vi "Drive_SetMotorsPosition.vi"(7 "ControlMode (CAN)":T1, 8 "error in (no error)":errorcluster, 9 "Distance Right":dbl, 10 "Distance Left":dbl) -> (0 "error out":errorcluster, 1 "Distance Right out":dbl, 2 "Distance Left out":dbl)   [LabVIEW 2009, in "Drive.lvlib"]
uses:
  Drive.lvlib
  Drive_ControlMode.ctl
  CAN/SubVIs/CAN Jaguar Control Mode.ctl
  OWNCAN.lvlib
  CAN.lvlib
  Drive_Utils.lvlib
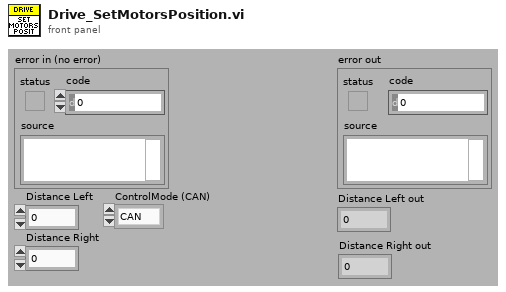
[diagram p1: front panel]
types:
  T1 = typedef "Drive.lvlib/Drive_ControlMode.ctl" = enum16{"CAN", "PWM"}
  T2 = typedef "CAN.lvlib/CAN Jaguar Control Mode.ctl" = enum16{"Percent VBus", "Speed", "Position", "Current"}
  T3 = typedef "Semaphore RefNum" = refnum<k1>
  T4 = cluster{"CAN Jaguar Ref Left":cluster{"Device Number":u8, "Control Mode":enum16{"Percent VBus", "Speed", "Position", "Current"}, "Inverted":bool, "Semaphore":T3, "Max Vout":dbl, "DevStatus":errorcluster}, "CAN Jaguar Ref Right":cluster{"Device Number":u8, "Control Mode":enum16{"Percent VBus", "Speed", "Position", "Current"}, "Inverted":bool, "Semaphore":T3, "Max Vout":dbl, "DevStatus":errorcluster}}
  T5 = enum16{"Percent VBus", "Speed", "Position", "Current"}
  T6 = typedef "OWNCAN.lvlib/CAN Jaguars Ref.ctl" = cluster{"CAN Jaguar Ref Left":T7, "CAN Jaguar Ref Right":T7}
  T7 = typedef "CAN.lvlib/CAN Jaguar Ref.ctl" = cluster{"Device Number":u8, "Control Mode":T2, "Inverted":bool, "Semaphore":T3, "Max Vout":dbl, "DevStatus":errorcluster}
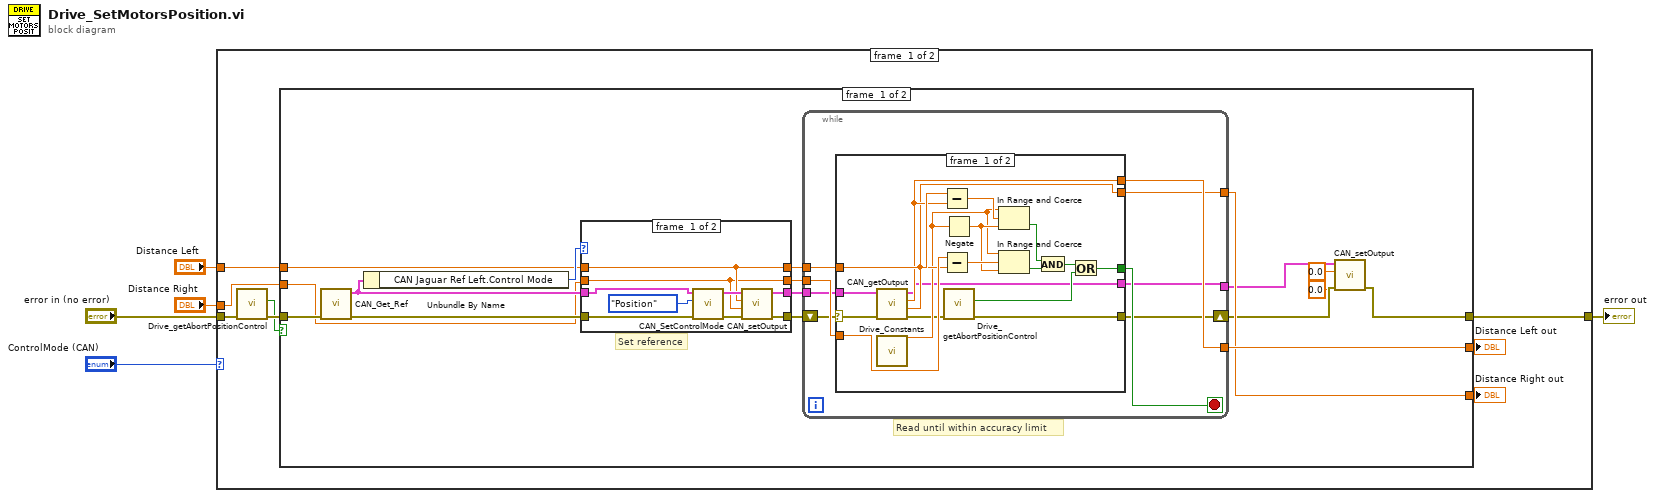
[diagram p0: block diagram]
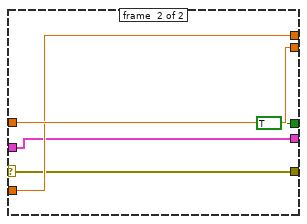
[diagram p2: hidden frame]
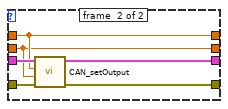
[diagram p3: hidden frame]
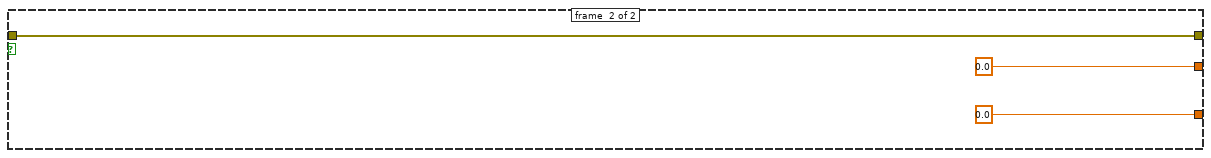
[diagram p4: hidden frame]
diagram:
  n1 = case shown="\"CAN\", Default" "ControlMode (CAN)" {
    tunnel: "error in (no error)" -> [w8 w81]
    tunnel: [w9 w81] -> w3
    tunnel: "Distance Left" -> [w13 _]
    tunnel: "Distance Right" -> [w12 _]
    frame #0 {
      n2 = call "Drive_getAbortPositionControl.vi"("error in (no error)"=w8) -> ("error out"=w7:errorcluster, "Abort Position Control"=w6:bool)  [unwired: 9 in]
      n3 = case shown="False" w6 {
        tunnel: w7 -> [w30 w80]
        tunnel: w13 -> [w26 _]
        tunnel: w12 -> [w25 _]
        tunnel: [w20 0.0 ("Left output")] -> w11
        tunnel: [w19 0.0 ("Right output")] -> w10
        tunnel: [w16 w80] -> w9
        frame #0 {
          # "Read until within accuracy limit"
          # "Set reference"
          n4 = call "CAN_Get_Ref.vi"("error in (no error)"=w30) -> ("error out"=w27:errorcluster, "CAN_Jaguars_ref"=w28:T4)  [unwired: 9 in]
          n5 = Unbundle By Name(w28) -> ("CAN Jaguar Ref Left.Control Mode"=w29:T5)
          n6 = case shown="Default" w29 {
            tunnel: w28 -> [w71 w77]
            tunnel: w27 -> [w68 w76]
            tunnel: [w66 w75] -> w24
            tunnel: w26 -> [w64 w73]
            tunnel: w25 -> [w63 w72]
            tunnel: [w65 w74] -> w23
            tunnel: [w64 w73] -> w22
            tunnel: [w63 w72] -> w21
            frame #0 {
              n7 = call "CAN_SetControlMode.vi"("error in (no error)"=w68, "Control Mode"=CAN_Jaguar_Control_Mode."Position", "CAN Jaguars Ref"=w71) -> ("error out"=w67:errorcluster, "CAN Jaguars Ref out"=w70:T6)  [unwired: 7 in]
              n8 = call "CAN_setOutput.vi"("error in (no error)"=w67, "Output Right"=w63, "Output Left"=w64, "CAN Jaguars Ref"=w70) -> ("error out"=w66:errorcluster, "CAN Jaguars Ref out"=w65:T6)  [unwired: 6 in]
            }
            frame #1 {
              n9 = call "CAN_setOutput.vi"("error in (no error)"=w76, "Output Right"=w72, "Output Left"=w73, "CAN Jaguars Ref"=w77) -> ("error out"=w75:errorcluster, "CAN Jaguars Ref out"=w74:T6)  [unwired: 6 in]
            }
          }
          n10 = while {
            tunnel: w23 -> [w37]
            tunnel: w22 -> [w39]
            tunnel: w21 -> [w38]
            shift-right: [w32] -> w17
            shift-left: w24 -> [w36]
            tunnel: [w34] -> w20
            tunnel: [w33] -> w19
            tunnel: [w31] -> w18
            stop <- w35 stop-if-true
            n11 = case shown="No Error" w36 {
              selector: w36 -> [w41 w60]
              tunnel: w37 -> [w57 w58]
              tunnel: w39 -> [w56 w62]
              tunnel: w38 -> [w55 w61]
              tunnel: [w50 w61] -> w34
              tunnel: [w49 w62] -> w33
              tunnel: [w45 w60] -> w32
              tunnel: [w42 TRUE] -> w35
              tunnel: [w40 w58] -> w31
              frame #0 {
                n12 = call "CAN_getOutput.vi"("error in (no error)"=w41, "CAN Jaguars Ref"=w57) -> ("error out"=w46:errorcluster, "Right output"=w49:dbl, "Left output"=w50:dbl, "CAN Jaguars Ref out"=w40:T6)  [unwired: 6 in]
                n13 = call "Drive_Constants.vi"() -> ("Position accuracy (m)"=w47:dbl)  [unwired: 20 in, 7 out]
                n14 = Subtract(x=w56, y=w50) -> (x-y=w54:dbl)
                n15 = Subtract(x=w55, y=w49) -> (x-y=w53:dbl)
                n16 = Negate(x=w47) -> (-x=w48:dbl)
                n17 = call "Drive_getAbortPositionControl.vi"("error in (no error)"=w46) -> ("error out"=w45:errorcluster, "Abort Position Control"=w43:bool)  [unwired: 9 in]
                n18 = In Range and Coerce(upper limit=w47, x=w54, lower limit=w48) -> (In Range?=w52:bool)  [unwired: 1 out]
                n19 = In Range and Coerce(upper limit=w47, x=w53, lower limit=w48) -> (In Range?=w51:bool)  [unwired: 1 out]
                n20 = And(x=w52, y=w51) -> (x .and. y?=w44:bool)
                n21 = Or(x=w44, y=w43) -> (x .or. y?=w42:bool)
              }
              frame #1 {
              }
            }
          }
          n22 = call "CAN_setOutput.vi"("error in (no error)"=w17, "Output Right"=0.0, "Output Left"=0.0, "CAN Jaguars Ref"=w18) -> ("error out"=w16:errorcluster)  [unwired: 6 in, 1 out]
        }
        frame #1 {
        }
      }
      "Distance Left out" <- w11
      "Distance Right out" <- w10
    }
    frame #1 {
      # "Not implemented"
    }
  }
  "error out" <- w3
